vi "View.vi"(8 "error in (no error)":errorcluster, 11 "Thermal Chamber Controller In":refnum<class "Thermal Chamber Controller.lvclass">) -> (0 "error out":errorcluster, 3 "Thermal Chamber Controller Out":refnum<class "Thermal Chamber Controller.lvclass">)   [LabVIEW 2020, in "Thermal Chamber Controller.lvclass"]
doc: "This VI implements the main UI of the process. A reference to this VI should be set using the Set View VI Reference.vi method when the VI is started."
uses:
  Thermal Chamber Controller.lvclass
  C:/Program Files (x86)/National Instruments/LabVIEW 2020/vi.lib/Asteme/Triarc Framework/Process/Process.lvclass
  C:/Program Files (x86)/National Instruments/LabVIEW 2020/vi.lib/Asteme/Triarc Framework/View/View.lvclass
  <vilib>/Asteme/Triarc Framework/View/View.lvclass/View.ctl
  Thermal Chamber Controller.lvclass/Thermal Chamber Controller.ctl
  Private/Heater State.ctl
  <vilib>/Asteme/Triarc Framework/View/View.lvclass
  <vilib>/Asteme/Triarc Framework/Process/Process.lvclass
  C:/Program Files (x86)/National Instruments/LabVIEW 2020/vi.lib/Asteme/Triarc Framework/Base/Base.lvclass
  C:/Program Files (x86)/National Instruments/LabVIEW 2020/vi.lib/Asteme/Triarc Framework/Error Handler Interface/Error Handler Interface.lvclass
  C:/Program Files (x86)/National Instruments/LabVIEW 2020/vi.lib/Asteme/Triarc Framework/Logging/Logging.lvclass
  C:/Users/anton/Documents/GitHub/Triarc-Examples/Thermal Chamber/Thermal Chamber Controller/Thermal Chamber Controller.lvclass
  C:/Program Files (x86)/National Instruments/LabVIEW 2020/vi.lib/Asteme/Triarc Framework/Helper Loop/Helper Loop.lvclass
panel:
  in  "Enable Heater":bool
  in  "Disable Heater":bool
  in  "Ramp Rate (deg C / second)":dbl=1.0
  in  "Temperature Set Point (deg C)":dbl=22.0
  out "Heater State":bool
  out "Actual Temperature":dbl format="%.2f"
  out "Chamber Temperature Chart":T1(graph)
  out "Status":string
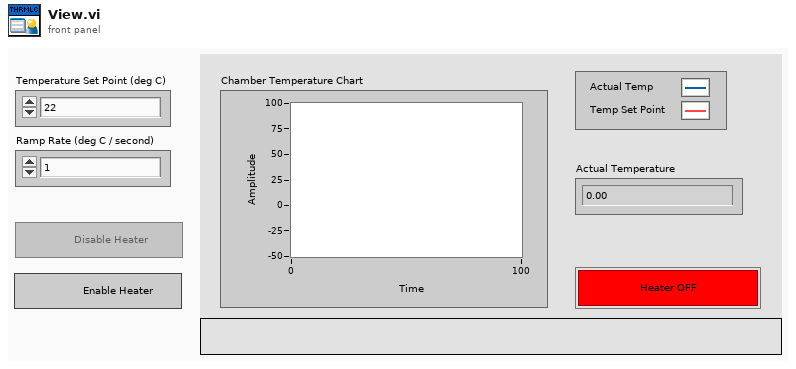
[diagram p1: front panel]
types:
  T1 = cluster{"Actual Temperature":dbl, "Required Temperature deg C":dbl}
  T2 = typedef "Thermal Chamber Controller.lvclass/Heater State.ctl" = enum16{"Heater Disabled", "Heater Enabled"}
  T3 = cluster{"Actual Temperature":dbl, "Temperature Set Point":dbl}
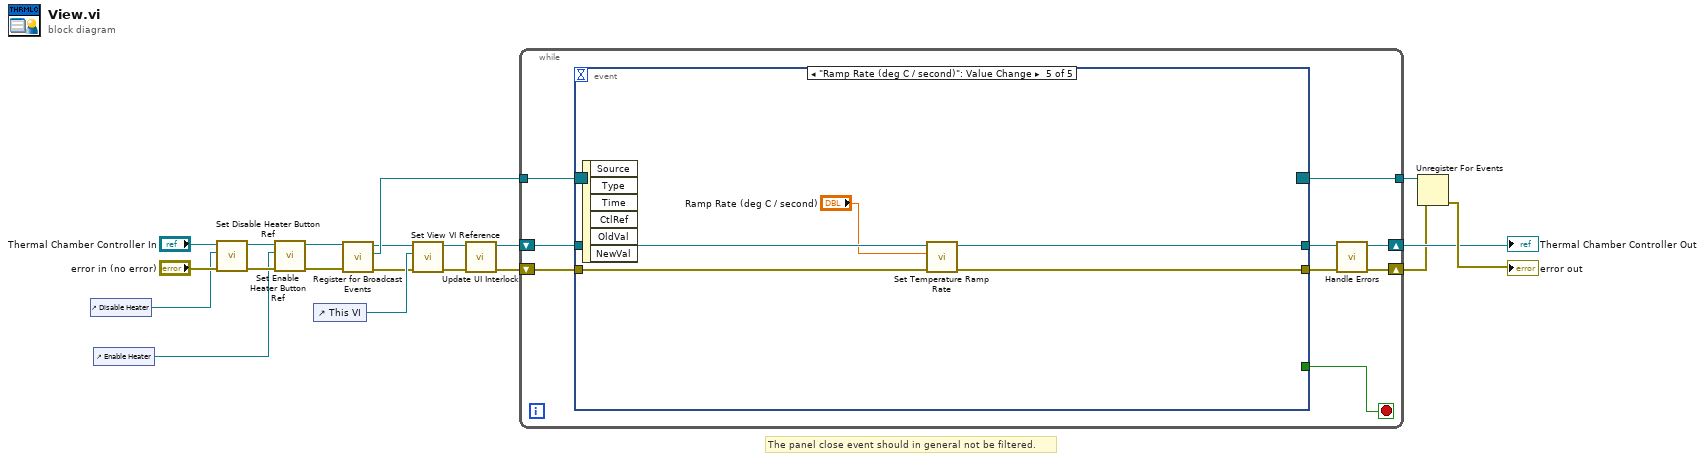
[diagram p0: block diagram]
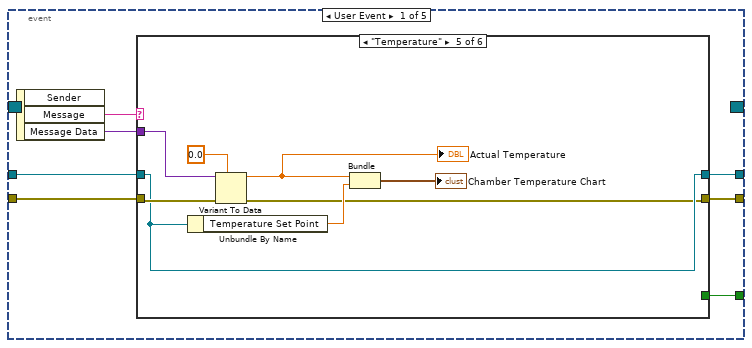
[diagram p2: hidden frame]
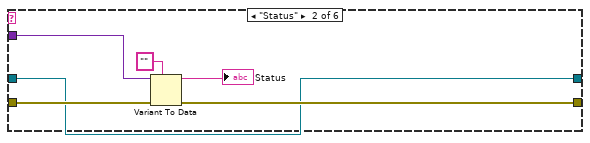
[diagram p4: hidden frame]
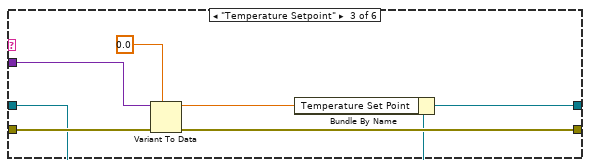
[diagram p5: hidden frame]
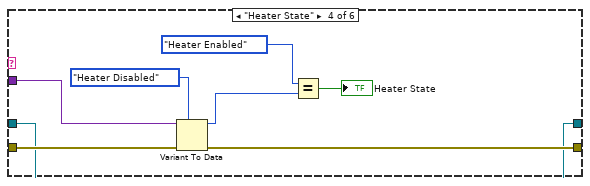
[diagram p6: hidden frame]
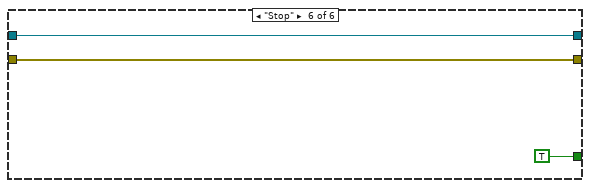
[diagram p7: hidden frame]
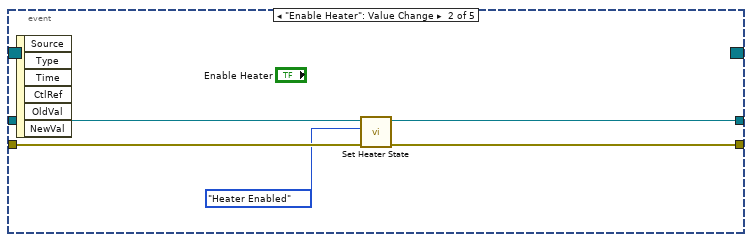
[diagram p8: hidden frame]
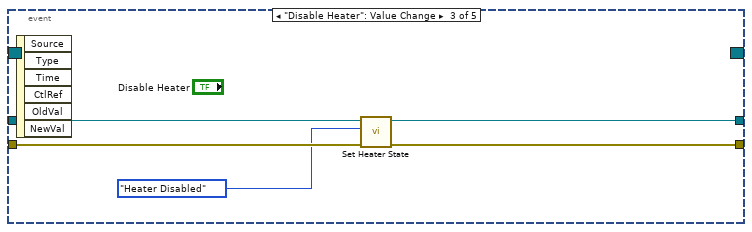
[diagram p9: hidden frame]
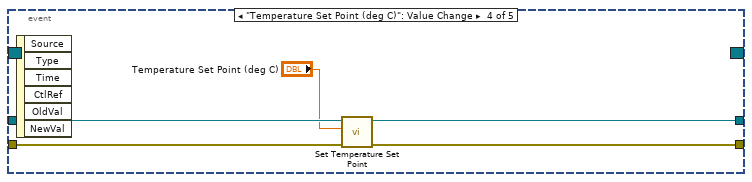
[diagram p10: hidden frame]
diagram:
  # "The panel close event should in general not be filtered."
  n1 = control-ref of="Disable Heater"() -> (w5:refnum<vi>)
  n2 = control-ref of="Enable Heater"() -> (w4:refnum<vi>)
  n3 = call "Set Disable Heater Button Ref.vi"("error in (no error)"="error in (no error)", "Disable Heater Button Ref"=w5, "Thermal Chamber Controller In"="Thermal Chamber Controller In") -> ("error out"=w8:errorcluster, "Thermal Chamber Controller Out"=w6:refnum<class "Thermal Chamber Controller.lvclass">)  [unwired: 7 in]
  n4 = call "Set Enable Heater Button Ref.vi"("error in (no error)"=w8, "Enable Heater Button Ref"=w4, "Thermal Chamber Controller In"=w6) -> ("error out"=w10:errorcluster, "Thermal Chamber Controller Out"=w9:refnum<class "Thermal Chamber Controller.lvclass">)  [unwired: 7 in]
  n5 = control-ref of="This VI"() -> (w17:refnum<vi>)
  n6 = call <vilib>:"Register for Broadcast Events.vi"("error in (no error)"=w10, "Process In"=w9) -> ("error out"=w15:errorcluster, "Event Registration Refnum Out"=w16:refnum<event-registration>, "Process Out"=w14:refnum<class "Thermal Chamber Controller.lvclass">)  [unwired: 7 in]
  n7 = call <vilib>:"Set View VI Reference.vi"("error in (no error)"=w15, "View VI Reference"=w17, "UI View in"=w14) -> ("error out"=w13:errorcluster, "UI View out"=w2:refnum<class "Thermal Chamber Controller.lvclass">)  [unwired: 7 in]
  n8 = call "Update UI Interlock.vi"("error in (no error)"=w13, "Thermal Chamber Controller In"=w2) -> ("error out"=w3:errorcluster, "Thermal Chamber Controller Out"=w1:refnum<class "Thermal Chamber Controller.lvclass">)  [unwired: 8 in]
  n9 = while {
    shift-right: [w23] -> w19
    shift-left: w1 -> [w29]
    shift-right: [w21] -> w12
    shift-left: w3 -> [w27]
    tunnel: w16 -> [w26]
    tunnel: [w25] -> w11
    stop <- w24 stop-if-true
    n10 = event shown="[4] \"Ramp Rate (deg C / second)\": Value Change" {
      selector: w26 -> [_ _ _ _ _]
      dyn-events: [_ _ _ _ _] -> w25
      timeout: _ -> [_ _ _ _ _]
      tunnel: w29 -> [w36 w73 w78 w85 w88]
      tunnel: [w35 w72 w77 w84 w87] -> w28
      tunnel: w27 -> [w33 w75 w80 w82 w90]
      tunnel: [w34 w74 w79 w83 w89] -> w22
      tunnel: [w31 _ _ _ _] -> w24
      event User Event {
        n11 = event-data() -> ("Message"=w32:string, "Message Data"=w30:variant)  [unwired: 1 in, 1 out]
        n12 = case shown="\"Temperature\"" w32 {
          tunnel: w36 -> [w38 w39 w48 w52 w62 w70]
          tunnel: [w38 w39 w46 w52 w62 w70] -> w35
          tunnel: [w37 w40 w49 w56 w61 w69] -> w34
          tunnel: w33 -> [w37 w43 w50 w57 w67 w69]
          tunnel: [_ _ _ _ _ TRUE] -> w31
          tunnel: w30 -> [_ w44 w51 w58 w66 _]
          frame Default {
          }
          frame "Status" {
            n13 = Variant To Data(error in=w43, type="", Variant=w44) -> (data=→"Status":string, error out=w40:errorcluster)
          }
          frame "Temperature Setpoint" {
            n14 = Variant To Data(error in=w50, type=0.0 ("Numeric"), Variant=w51) -> (data=w45:dbl, error out=w49:errorcluster)
            n15 = Bundle By Name(cluster=w48, "Temperature Set Point"=w45) -> (w46:refnum<class "Thermal Chamber Controller.lvclass">)
          }
          frame "Heater State" {
            n16 = Variant To Data(error in=w57, type=Heater_State."Heater Disabled" ("Heater State"), Variant=w58) -> (data=w54:T2, error out=w56:errorcluster)
            n17 = Equal?(x=Heater_State."Heater Enabled" ("Heater State"), y=w54) -> (x = y?=→"Heater State":bool)
          }
          frame "Temperature" {
            n18 = Unbundle By Name(w62) -> ("Temperature Set Point"=w63:dbl)
            n19 = Variant To Data(error in=w67, type=0.0 ("Actual Temperature"), Variant=w66) -> (data=w64:dbl, error out=w61:errorcluster)
            "Actual Temperature" <- w64
            n20 = Bundle("Actual Temperature"=w64, "Temperature Set Point"=w63) -> (→"Chamber Temperature Chart":T3)  [unwired: 1 in]
          }
          frame "Stop" {
          }
        }
      }
      event "Enable Heater": Value Change {
        n21 = event-data() -> ()  [unwired: 1 in, 6 out]
        n22 = call "Set Heater State.vi"("error in (no error)"=w75, "Heater State"=Heater_State."Heater Enabled", "Thermal Chamber Controller In"=w73) -> ("error out"=w74:errorcluster, "Thermal Chamber Controller Out"=w72:refnum<class "Thermal Chamber Controller.lvclass">)  [unwired: 7 in]
      }
      event "Disable Heater": Value Change {
        n23 = event-data() -> ()  [unwired: 1 in, 6 out]
        n24 = call "Set Heater State.vi"("error in (no error)"=w80, "Heater State"=Heater_State."Heater Disabled", "Thermal Chamber Controller In"=w78) -> ("error out"=w79:errorcluster, "Thermal Chamber Controller Out"=w77:refnum<class "Thermal Chamber Controller.lvclass">)  [unwired: 7 in]
      }
      event "Temperature Set Point (deg C)": Value Change {
        n25 = event-data() -> ()  [unwired: 1 in, 6 out]
        n26 = call "Set Temperature Set Point.vi"("error in (no error)"=w82, "Temperature Set Point"="Temperature Set Point (deg C)", "Thermal Chamber Controller In"=w85) -> ("error out"=w83:errorcluster, "Thermal Chamber Controller Out"=w84:refnum<class "Thermal Chamber Controller.lvclass">)  [unwired: 7 in]
      }
      event "Ramp Rate (deg C / second)": Value Change {
        n27 = event-data() -> ()  [unwired: 1 in, 6 out]
        n28 = call "Set Temperature Ramp Rate.vi"("error in (no error)"=w90, "Temperature Ramp Rate [degC/s]"="Ramp Rate (deg C / second)", "Thermal Chamber Controller In"=w88) -> ("error out"=w89:errorcluster, "Thermal Chamber Controller Out"=w87:refnum<class "Thermal Chamber Controller.lvclass">)  [unwired: 7 in]
      }
    }
    n29 = call-dynamic "Handle Errors.vi"("error in (no error)"=w22, "Process In"=w28) -> ("error out"=w21:errorcluster, "Process Out"=w23:refnum<class "Thermal Chamber Controller.lvclass">)  [unwired: 8 in]
  }
  "Thermal Chamber Controller Out" <- w19
  n30 = Unregister For Events(event registration refnum=w11, error in=w12) -> (error out=→"error out":errorcluster)
